vi "core_loop_timeout.vi"(9 "i (reset @ 0)":i32=1, 10 "timeout (2k ms)":i32=2000) -> (2 "timeout":bool, 3 "remaining time":i32)   [LabVIEW 2015]
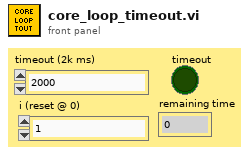
[diagram p1: front panel]
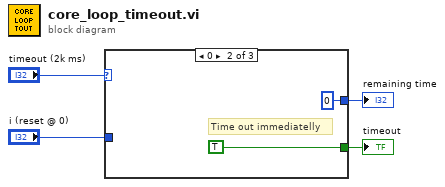
[diagram p0: block diagram]
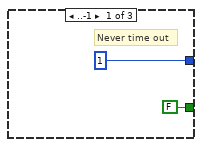
[diagram p2: hidden frame]
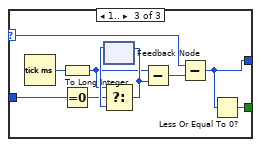
[diagram p3: hidden frame]
diagram:
  n1 = case shown="0" "timeout (2k ms)" {
    selector: "timeout (2k ms)" -> [_ _ w10]
    tunnel: [1 0 w15] -> w4
    tunnel: [FALSE TRUE w12] -> w3
    tunnel: "i (reset @ 0)" -> [_ _ w11]
    frame ..-1 {
      # "Never time out"
    }
    frame 0 {
      # "Time out immediatelly"
    }
    frame 1.. {
      n2 = Tick Count (ms) ("now")() -> (millisecond timer value=w14:u32)
      n3 = To Long Integer(number=w14) -> (32bit integer=w13:i32)
      n4 = Equal To 0?(x=w11) -> (x = 0?=w9:bool)
      n5 = feedback #1() -> (w18:i32)  [unwired: 1 in]
      n6 = Select(t=w13, s=w9, f=w18) -> (s? t:f=w17:i32)
      n7 = feedback-in #1(w17) -> ()
      n8 = Subtract(x=w13, y=w17) -> (x-y=w16:i32)
      n9 = Subtract(x=w10, y=w16) -> (x-y=w15:i32)
      n10 = Less Or Equal To 0?(x=w15) -> (x <= 0?=w12:bool)
    }
  }
  "timeout" <- w3
  "remaining time" <- w4
